vi "gcode.vi"() -> ()   [LabVIEW 2020]
uses:
  bee2abb7-c490-4ad6-bfc0-30ed72578e14.vi
panel:
  in  "Gcode":string
  out "Array":cluster{"x":dbl, "y":dbl}[](array[cluster])
  out "XY Graph":cluster{dbl[], dbl[]}(graph)
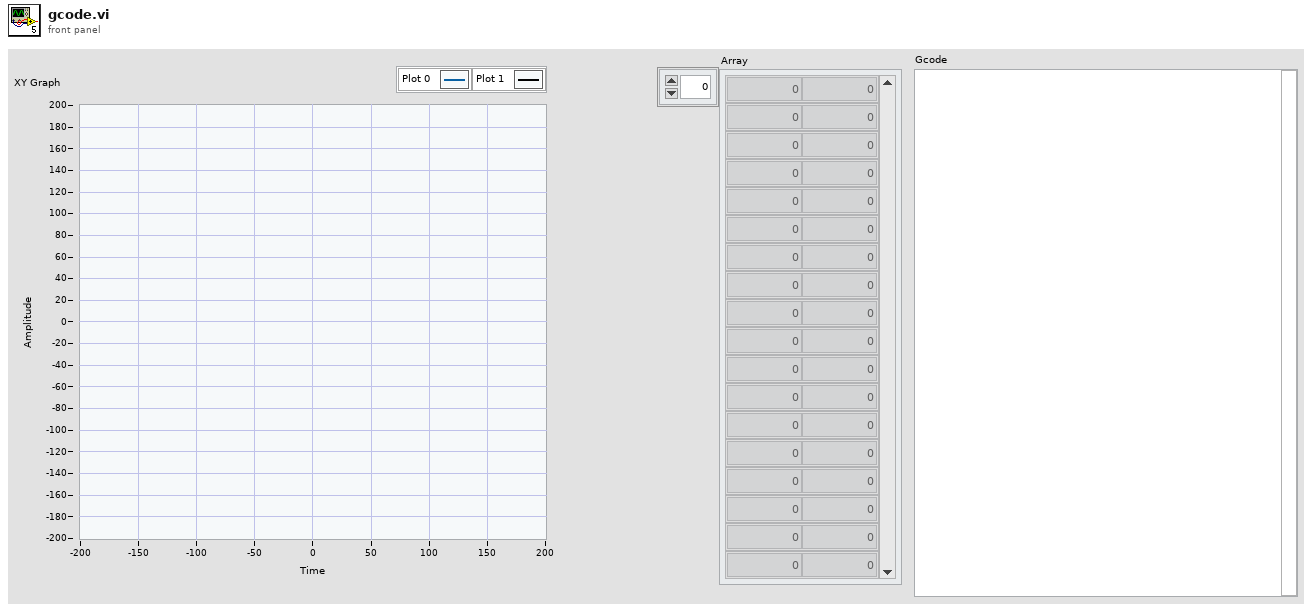
[diagram p1: front panel]
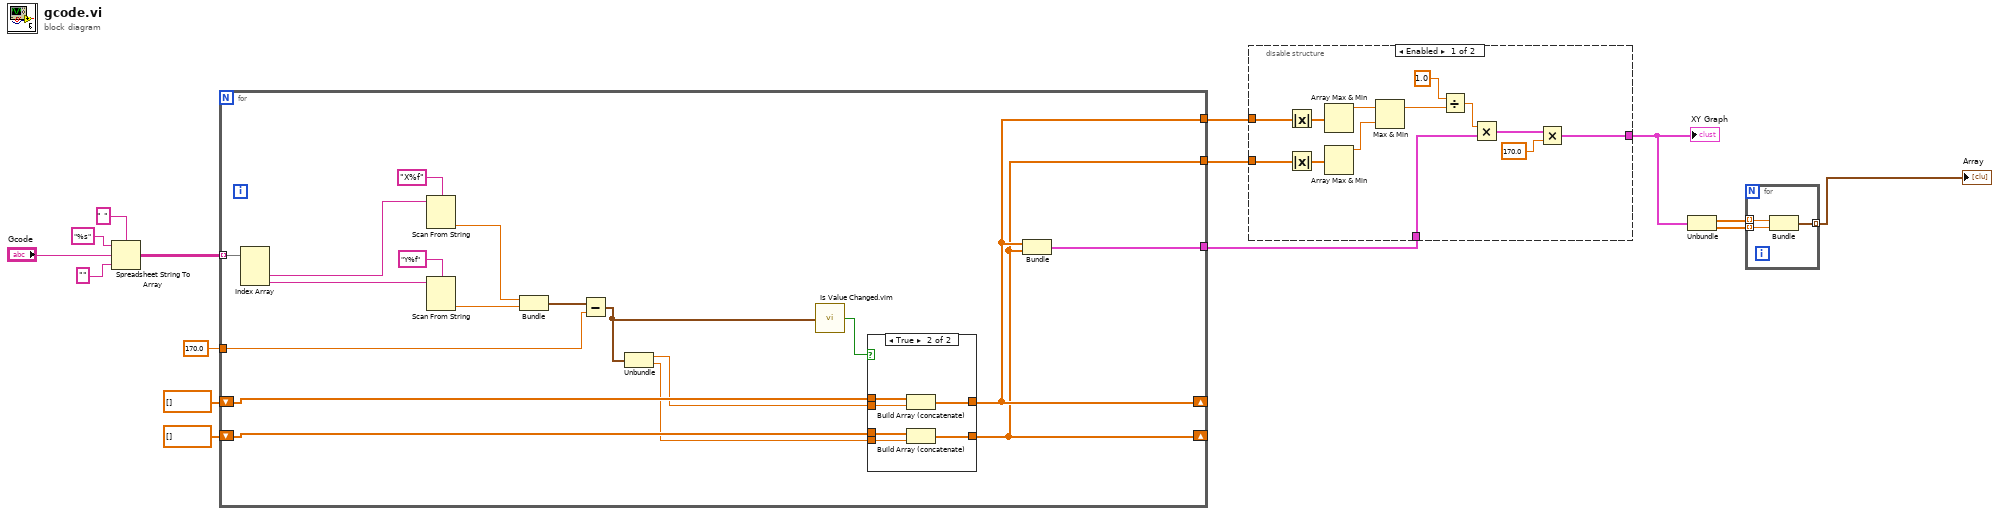
[diagram p0: block diagram]
diagram:
  n1 = Spreadsheet String To Array(delimiter (Tab)=" ", format string="%s", spreadsheet string="Gcode", array type (2D Dbl)="" ("delimiter (Tab)")) -> (array=w2:string[][])
  n2 = for {
    shift-right: [w29] -> _
    shift-left: dbl[] [] -> [w32]
    shift-right: [w28] -> _
    shift-left: dbl[] [] -> [w31]
    tunnel: [w30] -> w11
    tunnel: [w29] -> w13
    tunnel: [w28] -> w12
    tunnel: w2 -> [w24] mode=indexing
    tunnel: 170.0 -> [w19]
    n3 = Index Array(array=w24) -> (element #2=w23:string, element #3=w22:string)  [unwired: 3 in, 1 out]
    n4 = Scan From String(format string="X%f", input string=w23) -> (output 1=w26:dbl)  [unwired: 3 in, 3 out]
    n5 = Scan From String(format string="Y%f", input string=w22) -> (output 1=w21:dbl)  [unwired: 3 in, 3 out]
    n6 = Bundle(w26, w21) -> (w20:cluster{dbl, dbl})  [unwired: 1 in]
    n7 = Subtract(x=w20, y=w19) -> (x-y=w18:cluster{dbl, dbl})
    n8 = Unbundle(w18) -> (w17:dbl, w16:dbl)
    n9 = call "Is Value Changed.vim"("value"=w18) -> ("changed or first call?"=w33:bool)
    n10 = case shown="True" w33 {
      tunnel: w17 -> [_ w41]
      tunnel: w16 -> [_ w40]
      tunnel: [w35 w39] -> w29
      tunnel: [w34 w38] -> w28
      tunnel: w32 -> [w35 w37]
      tunnel: w31 -> [w34 w36]
      frame False {
      }
      frame True {
        n11 = Build Array (concatenate)(w37, w41) -> (w39:dbl[])
        n12 = Build Array (concatenate)(w36, w40) -> (w38:dbl[])
      }
    }
    n13 = Bundle(w29, w28) -> (w30:cluster{dbl[], dbl[]})  [unwired: 1 in]
  }
  n14 = disable-structure shown="Enabled" {
    disable-tunnel: w13 -> [w54 _]
    disable-tunnel: w12 -> [w53 _]
    disable-tunnel: w11 -> [w45 w55]
    disable-tunnel: [w42 w55] -> w10
    frame Enabled {
      n15 = Absolute Value(x=w54) -> (abs(x)=w52:dbl[])
      n16 = Absolute Value(x=w53) -> (abs(x)=w51:dbl[])
      n17 = Array Max & Min(array=w52) -> (max value=w50:dbl)  [unwired: 3 out]
      n18 = Array Max & Min(array=w51) -> (max value=w49:dbl)  [unwired: 3 out]
      n19 = Max & Min(x=w50, y=w49) -> (max(x,y)=w48:dbl)  [unwired: 1 out]
      n20 = Divide(x=1.0, y=w48) -> (x/y=w46:dbl)
      n21 = Multiply(x=w46, y=w45) -> (x*y=w44:cluster{dbl[], dbl[]})
      n22 = Multiply(x=w44, y=170.0 ("x")) -> (x*y=w42:cluster{dbl[], dbl[]})
    }
    frame Disabled {
    }
  }
  "XY Graph" <- w10
  n23 = Unbundle(w10) -> (w9:dbl[], w8:dbl[])
  n24 = for {
    tunnel: w9 -> [w58] mode=indexing
    tunnel: w8 -> [w57] mode=indexing
    tunnel: [w56] -> w7 mode=indexing
    n25 = Bundle("x"=w58, "y"=w57) -> (w56:cluster{"x":dbl, "y":dbl})  [unwired: 1 in]
  }
  "Array" <- w7
